vi "cmdLineParser_eventCpp.vi"(8 "error in (no error)":errorcluster, 11 "cmdLineArgs":string[](array[string])) -> (0 "error out":errorcluster, 1 "pathEventCpp":path, 2 "pathLvLib":path, 3 "pathMonitor":path, 5 "filesExist":bool)   [LabVIEW 2018]
doc: "Command line parser of getting/sending event to get the paths of SAL LabVIEW monitor, LvLib, and cpp file of getting/sending the event."
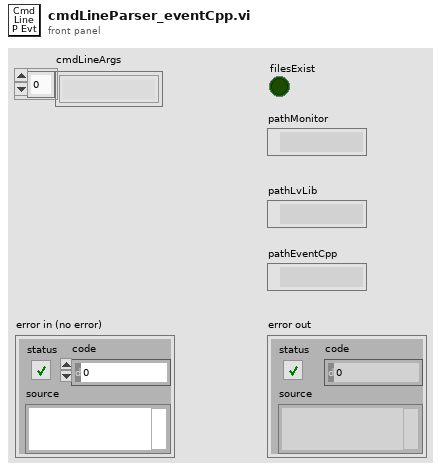
[diagram p1: front panel]
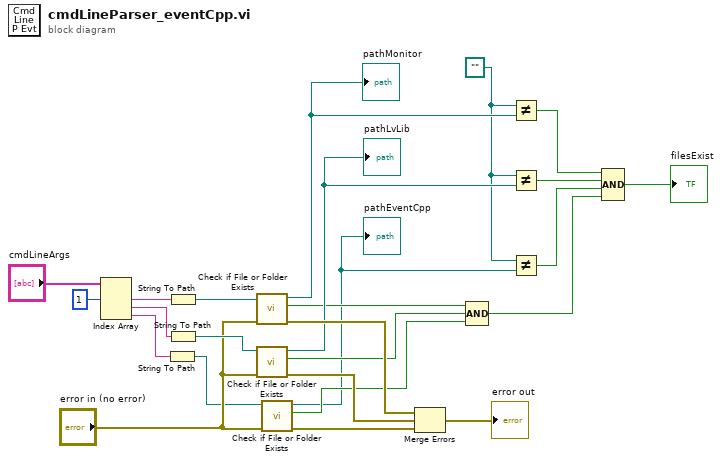
[diagram p0: block diagram]
diagram:
  w3 = path ""
  n1 = Index Array(array="cmdLineArgs", index #1=1 ("index")) -> (element #1=w24:string, element #2=w23:string, element #3=w10:string)  [unwired: 2 in]
  n2 = String To Path(string=w10) -> (path=w9:path)
  n3 = String To Path(string=w24) -> (path=w22:path)
  n4 = String To Path(string=w23) -> (path=w21:path)
  n5 = call <vilib>:"Check if File or Folder Exists.vi"("error in (no error)"="error in (no error)", "path"=w22) -> ("error out"=w20:errorcluster, "file or folder exists?"=w7:bool, "dup path"=w17:path)  [unwired: 7 in]
  "pathMonitor" <- w17
  n6 = call <vilib>:"Check if File or Folder Exists.vi"("error in (no error)"="error in (no error)", "path"=w21) -> ("error out"=w19:errorcluster, "file or folder exists?"=w6:bool, "dup path"=w16:path)  [unwired: 7 in]
  "pathLvLib" <- w16
  n7 = call <vilib>:"Check if File or Folder Exists.vi"("error in (no error)"="error in (no error)", "path"=w9) -> ("error out"=w8:errorcluster, "file or folder exists?"=w5:bool, "dup path"=w2:path)  [unwired: 7 in]
  "pathEventCpp" <- w2
  n8 = Merge Errors(w20, w19, w8) -> (→"error out":errorcluster)
  n9 = Compound Arithmetic op=AND(w7, w6, w5) -> (w4:bool)
  n10 = Not Equal?(x=w3, y=w17) -> (x != y?=w15:bool)
  n11 = Not Equal?(x=w3, y=w16) -> (x != y?=w14:bool)
  n12 = Not Equal?(x=w3, y=w2) -> (x != y?=w1:bool)
  n13 = Compound Arithmetic op=AND(w15, w14, w1, w4) -> (→"filesExist":bool)
